vi "nextfilename.vi"(11 "Path In":path) -> (3 "Incremented Path Out":path)   [LabVIEW 2020]
panel:
  # "This VI requires the filename have an underscore separating the name from the index for this VI to work correctly. For example, Filename_2.tmp would return Filename_3.tmp"
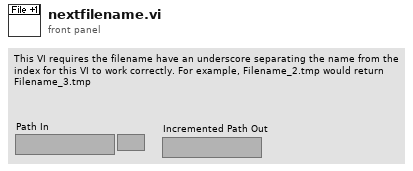
[diagram p1: front panel]
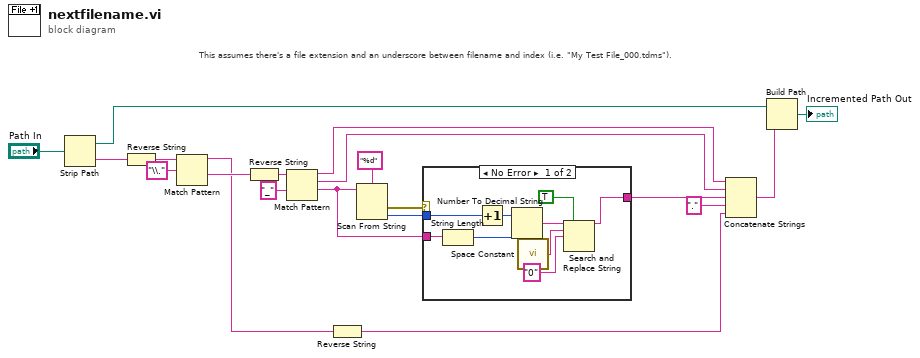
[diagram p0: block diagram]
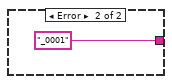
[diagram p2: hidden frame]
diagram:
  # "This assumes there's a file extension and an underscore between filename and index (i.e. \"My Test File_000.tdms\")."
  n1 = Strip Path(path="Path In") -> (stripped path=w1:path, name=w4:string)
  n2 = Reverse String(1:w4) -> (0:w19:string)
  n3 = Match Pattern(string=w19, regular expression="\\.") -> (before substring=w15:string, after substring=w17:string)  [unwired: 1 in, 2 out]
  n4 = Reverse String(1:w17) -> (0:w10:string)
  n5 = Match Pattern(string=w10, regular expression="_") -> (before substring=w8:string, match substring=w7:string, after substring=w6:string)  [unwired: 1 in, 1 out]
  n6 = Reverse String(1:w15) -> (0:w14:string)
  n7 = Scan From String(format string="%d", input string=w6) -> (error out=w12:errorcluster, output 1=w11:i32)  [unwired: 3 in, 2 out]
  n8 = case shown="No Error" w12 {
    tunnel: w11 -> [w22 _]
    tunnel: [w23 "_0001"] -> w20
    tunnel: w6 -> [w21 _]
    frame No Error {
      n9 = String Length(string=w21) -> (length=w28:i32)
      n10 = Increment(x=w22) -> (x+1=w29:i32)
      n11 = Number To Decimal String(number=w29, width (-)=w28) -> (decimal integer string=w27:string)
      n12 = call <vilib>:"Space Constant.vi"() -> ("String"=w25:string)
      n13 = Search and Replace String(replace all?=TRUE ("replace all? (F)"), input string=w27, search string=w25, replace string="0") -> (result string=w23:string)  [unwired: 4 in, 3 out]
    }
    frame Error {
    }
  }
  n14 = Concatenate Strings(w8, w7, w20, "." ("string"), w14) -> (w2:string)
  n15 = Build Path(base path=w1, name or relative path=w2) -> (appended path=→"Incremented Path Out":path)
